vi "Set Graph Samples.vi"(0 "reference in":refnum<class "Grapher.lvclass">, 2 "Graph Samples":u32, 5 "Error In":errorcluster) -> (14 "reference out":refnum<class "Grapher.lvclass">, 19 "Error Out":errorcluster)   [LabVIEW 2023, in "Grapher.lvclass"]
uses:
  Grapher.lvclass
  Grapher.lvclass/Grapher.ctl
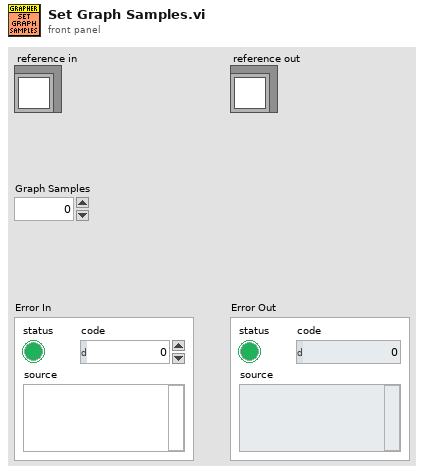
[diagram p1: front panel]
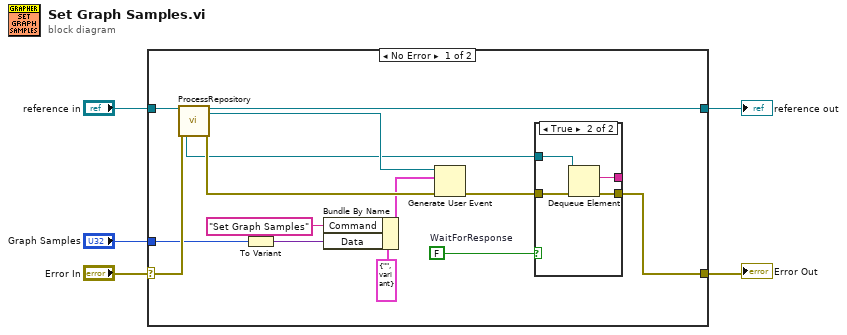
[diagram p0: block diagram]
diagram:
  n1 = case shown="No Error" "Error In" {
    selector: "Error In" -> [w19 w26]
    tunnel: [w12 w26] -> w4
    tunnel: [w17 w25] -> w2
    tunnel: "reference in" -> [w18 w25]
    tunnel: "Graph Samples" -> [w7 _]
    frame No Error {
      w15 = FALSE  # WaitForResponse
      n2 = call "ProcessRepository.vi"("reference in"=w18, "Error In"=w19) -> ("QueueFromProcess"=w9:refnum<queue>, "reference out"=w17:refnum<class "Grapher.lvclass">, "EventsToProcess"=w16:refnum<user-event>, "Error Out"=w13:errorcluster)  [unwired: 10 in, 4 out]
      n3 = To Variant(anything=w7) -> (Variant=w6:variant)
      n4 = Bundle By Name(cluster=cluster{"Command":string, "Data":variant} {"Command"="", "Data"=variant} ("MessageToProcess"), "Command"="Set Graph Samples", "Data"=w6) -> (w10:cluster{"Command":string, "Data":variant})
      n5 = Generate User Event(user event=w16, event data cluster=w10, error in=w13) -> (error out=w14:errorcluster)  [unwired: 1 in, 1 out]
      n6 = case shown="True" w15 {
        tunnel: w14 -> [w20 w24]
        tunnel: [_ w23] -> _
        tunnel: [w20 w22] -> w12
        tunnel: w9 -> [_ w21]
        frame False {
        }
        frame True {
          n7 = Dequeue Element(queue=w21, error in (no error)=w24) -> (element=w23:string, error out=w22:errorcluster)  [unwired: 1 in, 2 out]
        }
      }
    }
    frame Error {
    }
  }
  "Error Out" <- w4
  "reference out" <- w2
